vi "PTScanner.add object.vi"(0 "i ref in":refnum<vi>, 2 "Parameters":T1, 5 "error in (no error)":errorcluster) -> (14 "i ref out":refnum<vi>, 19 "error out":errorcluster)   [LabVIEW 2014, in "PTScanner.lvlib"]
uses:
  PTScanner.lvlib
  PTScanner.obj parameters.ctl
  CSlibraries-extern/DimLVEvent/LVDimInterface/LVDimInterface.lvlib
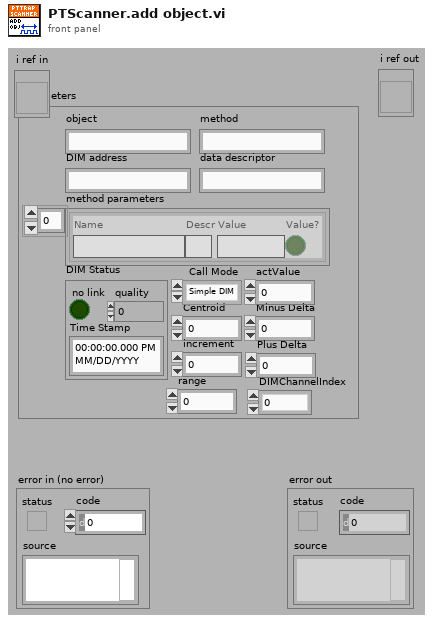
[diagram p1: front panel]
types:
  T1 = typedef "PTScanner.lvlib/PTScanner.obj parameters.ctl" = cluster{"object":string, "DIM address":string, "method":string, "data descriptor":string, "method parameters":cluster{"Name":string, "Descr":string, "Value":string, "Value?":bool}[], "Call Mode":enum16{"Simple DIM", "Synchronous"}, "actValue":dbl, "Centroid":dbl, "Minus Delta":dbl, "Plus Delta":dbl, "increment":dbl, "DIM Status":cluster{"no link":bool, "quality":i32, "Time Stamp":timestamp}, "range":dbl, "DIMChannelIndex":i32}
  T2 = typedef "PTScanner.lvlib/PTScanner.i attribute.ctl" = cluster{"Object cmds":T1[], "Steps":cluster{"Finished":bool, "cmd setup":T3[]}[], "curStep":i32, "DIM IDs":cluster{"AllFinished":i32, "Finished":i32, "curStep":i32, "nofSteps":i32, "NomValues":i32[], "1D-Min":i32, "1D-Max":i32, "Dimensions":i32, "MaxDimensions":i32, "ScanedDeviceNames":i32[]}, "All Finished":bool, "DIMs in use":string[], "Running":bool, "Scan Delay":u32, "loop":bool, "Paused":bool, "Formed":bool}
  T3 = typedef "PTScanner.lvlib/PTScanner.step obj parameters.ctl" = cluster{"obj index":i32, "nomValue":dbl, "fulfilled":bool}
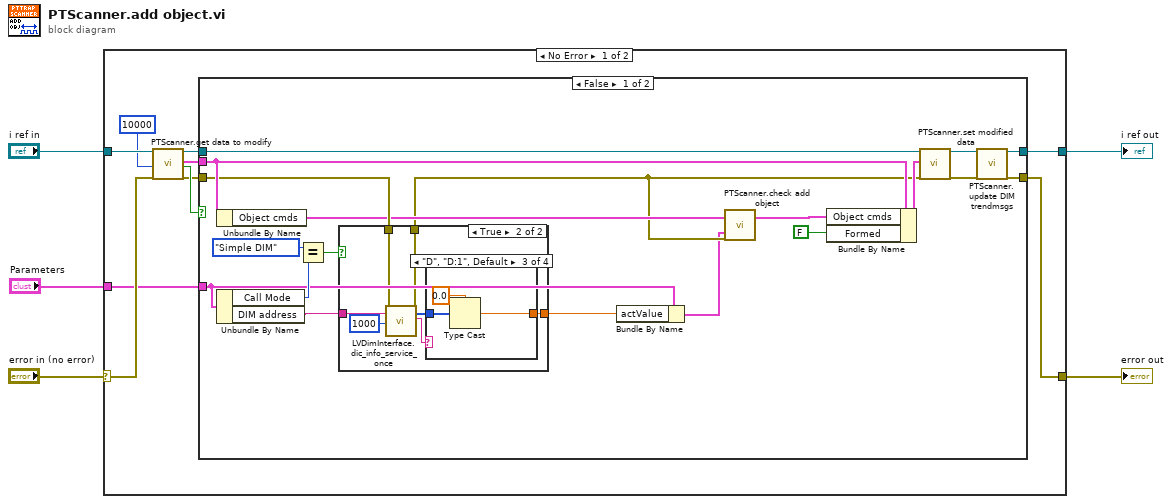
[diagram p0: block diagram]
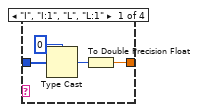
[diagram p3: hidden frame]
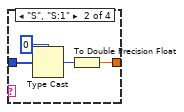
[diagram p4: hidden frame]
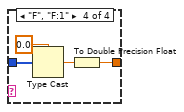
[diagram p5: hidden frame]
diagram:
  n1 = case shown="No Error" "error in (no error)" {
    selector: "error in (no error)" -> [w10 w60]
    tunnel: "i ref in" -> [w11 w61]
    tunnel: [w9 w61] -> w3
    tunnel: [w8 w60] -> w2
    tunnel: "Parameters" -> [w6 _]
    frame No Error {
      n2 = call "PTScanner.get data to modify.vi"("i ref in"=w11, "ms timeout (10000)"=10000, "error in (no error)"=w10) -> ("i ref out"=w14:refnum<vi>, "i attribute"=w12:T2, "timed out"=w15:bool, "error out"=w13:errorcluster)  [unwired: 13 in]
      n3 = case shown="False" w15 {
        tunnel: w14 -> [w34 w58]
        tunnel: w13 -> [w27 w59]
        tunnel: w12 -> [w33 _]
        tunnel: [w29 w59] -> w8
        tunnel: [w28 w58] -> w9
        tunnel: w6 -> [w17 _]
        frame False {
          n4 = Unbundle By Name(w33) -> ("Object cmds"=w23:T1[])
          n5 = Unbundle By Name(w17) -> ("Call Mode"=w18:enum16{"Simple DIM", "Synchronous"}, "DIM address"=w19:string)
          n6 = Equal?(x=enum16{"Simple DIM", "Synchronous"}."Simple DIM" ("Call Mode"), y=w18) -> (x = y?=w24:bool)
          n7 = case shown="True" w24 {
            tunnel: w19 -> [_ w41]
            tunnel: w27 -> [w35 w40]
            tunnel: [w35 w39] -> w21
            tunnel: [_ w36] -> w20
            frame False {
            }
            frame True {
              n8 = call "LVDimInterface.dic_info_service_once.vi"("serviceName"=w41, "timeout [ms]"=u32 1000, "error in (no error)"=w40) -> ("data"=w37:i8[], "typeDescriptor"=w38:string, "error out"=w39:errorcluster)  [unwired: 13 in, 1 out]
              n9 = case shown="\"D\", \"D:1\", Default" w38 {
                tunnel: w37 -> [w45 w49 w52 w56]
                tunnel: [w43 w47 w51 w54] -> w36
                frame "I", "I:1", "L", "L:1" {
                  n10 = Type Cast(type=0, x=w45) -> (*(type *) &x=w44:i32)
                  n11 = To Double Precision Float(number=w44) -> (double precision float=w43:dbl)
                }
                frame "S", "S:1" {
                  n12 = Type Cast(type=i16 0, x=w49) -> (*(type *) &x=w48:i16)
                  n13 = To Double Precision Float(number=w48) -> (double precision float=w47:dbl)
                }
                frame "D", "D:1", Default {
                  n14 = Type Cast(type=0.0, x=w52) -> (*(type *) &x=w51:dbl)
                }
                frame "F", "F:1" {
                  n15 = Type Cast(type=sgl 0.0, x=w56) -> (*(type *) &x=w55:sgl)
                  n16 = To Double Precision Float(number=w55) -> (double precision float=w54:dbl)
                }
              }
            }
          }
          n17 = Bundle By Name(cluster=w17, "actValue"=w20) -> (w16:T1)
          n18 = call "PTScanner.check add object.vi"("Object cmds"=w23, "new obj command"=w16, "error in (no error)"=w21) -> ("Object cmds out"=w22:T1[])  [unwired: 15 in, 1 out]
          n19 = Bundle By Name(cluster=w33, "Object cmds"=w22, "Formed"=FALSE) -> (w32:T2)
          n20 = call "PTScanner.set modified data.vi"("i ref in"=w34, "CLASS.i attribute"=w32, "error in (no error)"=w21) -> ("i ref out"=w30:refnum<vi>, "error out"=w31:errorcluster)  [unwired: 15 in]
          n21 = call "PTScanner.update DIM trendmsgs.vi"("i ref in"=w30, "error in"=w31) -> ("i ref out"=w28:refnum<vi>, "error out"=w29:errorcluster)  [unwired: 16 in]
        }
        frame True {
        }
      }
    }
    frame Error {
    }
  }
  "i ref out" <- w3
  "error out" <- w2
